vi "Synthesize.vi"(0 "Waveform in":refnum<class "Waveform.lvclass">, 5 "Fs (Hz)":dbl, 7 "Npts":i32, 9 "Repetition":i32, 11 "error in (no error)":errorcluster) -> (4 "Waveform out":refnum<class "Waveform.lvclass">, 8 "Array":dbl[](array[numeric]), 15 "error out":errorcluster)   [LabVIEW 2015, in "Waveform.lvclass"]
uses:
  Waveform.lvclass
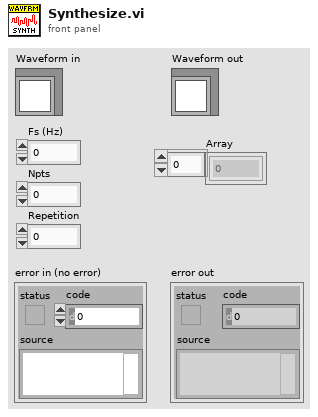
[diagram p1: front panel]
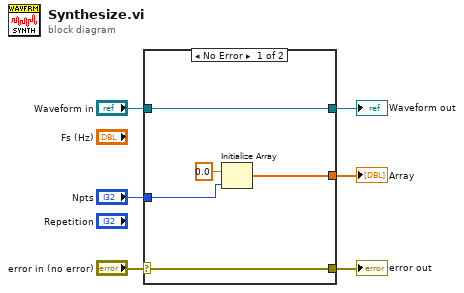
[diagram p0: block diagram]
diagram:
  n1 = case shown="No Error" "error in (no error)" {
    selector: "error in (no error)" -> [w10 w13]
    tunnel: [w10 w13] -> w5
    tunnel: [w11 w12] -> w3
    tunnel: "Waveform in" -> [w11 w12]
    tunnel: "Npts" -> [w8 _]
    tunnel: [w7 _] -> w1
    frame No Error {
      n2 = Initialize Array(0.0 ("element"), w8) -> (w7:dbl[])
    }
    frame Error {
    }
  }
  "error out" <- w5
  "Waveform out" <- w3
  "Array" <- w1
